vi "AR-31858A-Read-Anlog.vi"(8 "error in (no error)":errorcluster) -> (0 "error out":errorcluster, 3 "Registers":u16[](array[numeric]))   [LabVIEW 2016, in "环境动力监测库.lvlib" / "浮标电源管理.lvlib"]
uses:
  <vilib>/Plasmionique/MB Master/MB_Master/MB_Master.lvclass
  <vilib>/Plasmionique/MB Master/MB Master.lvlib
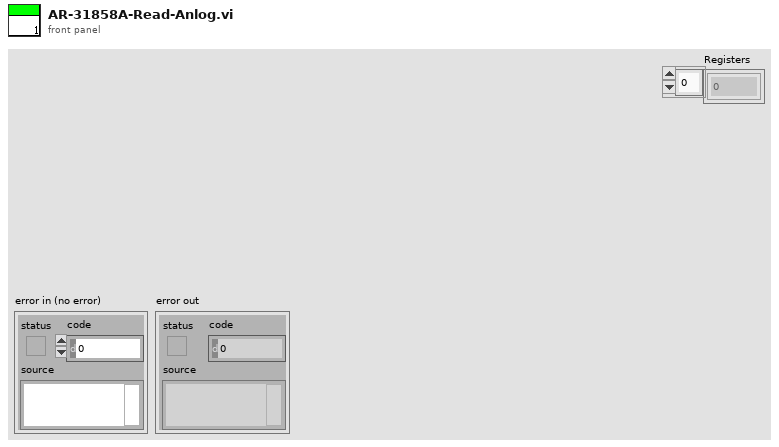
[diagram p1: front panel]
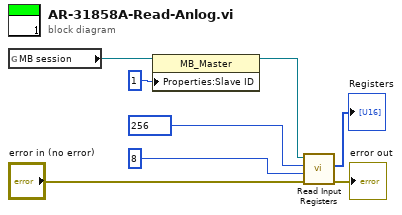
[diagram p0: block diagram]
diagram:
  n1 = global read "通讯全局变量.vi" "MB session"() -> (w4:refnum<class "MB_Master.lvclass">)
  n2 = property class="MB_Master"(reference=w4, "Properties:Slave ID"=u8 1 ("Slave ID")) -> (reference out=w3:refnum<class "MB_Master.lvclass">)  [unwired: 1 in, 1 out]
  n3 = call <vilib>:"Read Input Registers.vi"("error in (no error)"="error in (no error)", "quantity"=u16 8, "starting address"=u16 256, "MB session in"=w3) -> ("error out"=→"error out":errorcluster, "Registers"=→"Registers":u16[])  [unwired: 5 in, 1 out]
